vi "Initialize Hardware.vi"(8 "error in (no error)":errorcluster, 10 "Instruments":refnum<class "Instrument.lvclass">[](array[class]), 11 "Acro Template in":refnum<class "Example Application.lvclass">) -> (0 "error out":errorcluster, 3 "Acro Template out":refnum<class "Example Application.lvclass">)   [LabVIEW 2015, in "Example Application.lvlib" / "Example Application.lvclass"]
uses:
  Example Application.lvclass
  CBTF Modules/Classes/Instruments/Instrument/Class/Instrument.lvclass
  typedefs/Instrument Selector -- Enum.ctl
  CBTF Modules/Classes/Application/Class/Application.lvclass
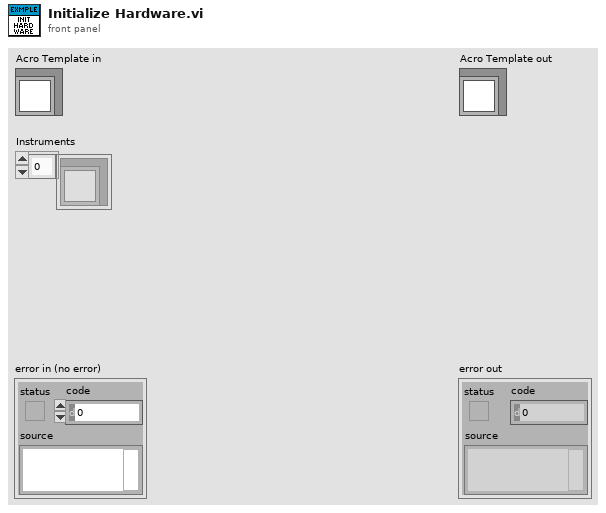
[diagram p1: front panel]
types:
  T1 = typedef "Example Application.lvlib/Example Application.lvclass/Instrument Selector -- Enum.ctl" = enum16{"AC Power Supply", "DC Power Supply 1"}
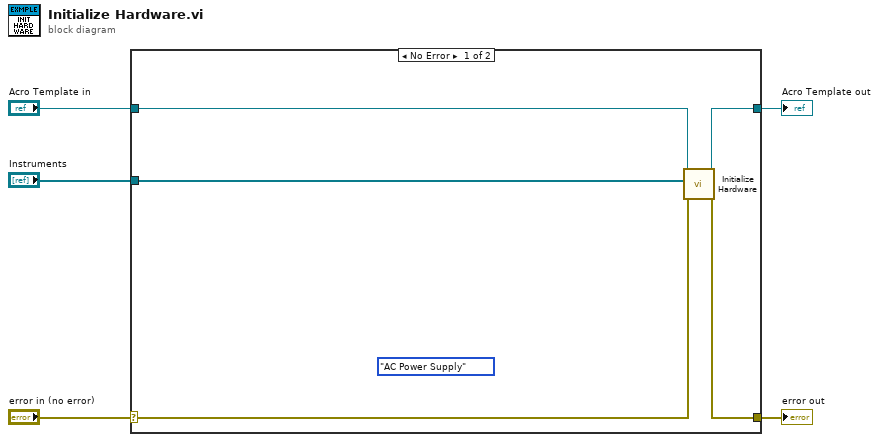
[diagram p0: block diagram]
diagram:
  n1 = case shown="No Error" "error in (no error)" {
    selector: "error in (no error)" -> [w8 w12]
    tunnel: [w7 w12] -> w4
    tunnel: [w9 w11] -> w2
    tunnel: "Acro Template in" -> [w10 w11]
    tunnel: "Instruments" -> [w6 _]
    frame No Error {
      (unwired) Instrument_Selector_--_Enum."AC Power Supply"
      n2 = call-parent "Initialize Hardware.vi"("error in (no error)"=w8, "Instruments"=w6, "Application in"=w10) -> ("error out"=w7:errorcluster, "Application out"=w9:refnum<class "Example Application.lvclass">)  [unwired: 7 in]
    }
    frame Error {
    }
  }
  "error out" <- w4
  "Acro Template out" <- w2
